vi "Arm Main.vi"() -> ()   [LabVIEW 2013]
doc: "This example shows how to move a motor connected to an encoder and a wheel, and then read information about the system from an encoder.\n\nThis is an example of how to use feedback (from the encoder) to create an open loop system. If some control method was used, for example using PID, a closed loop system could be created."
uses:
  <vilib>/Rock Robotics/WPI/DriverStation/WPI_DriverStationRobotMode2.ctl
  Robot Global Data.vi
panel:
  in  "Increment Down":dbl=-8.0
  in  "Increment Up":dbl=5.0
  in  "Incremented Angle":dbl=180.0
  in  "Biased Voltage":dbl=-0.5
  in  "Motor Upper Limit":dbl format="%#_13g"
  in  "Motor Lower Limit":dbl=-0.55 format="%#_13g"
  out "Arm Angle":dbl(graph)=177.5123200166945
  out "Motor Output":dbl(graph)
  in  "Arm Gain":dbl=0.01
  out "Arm Angle (deg)":dbl(knob)=177.5123200166945 scale=0.0..360.0 scale format="%#_3g"
  # "Output information."
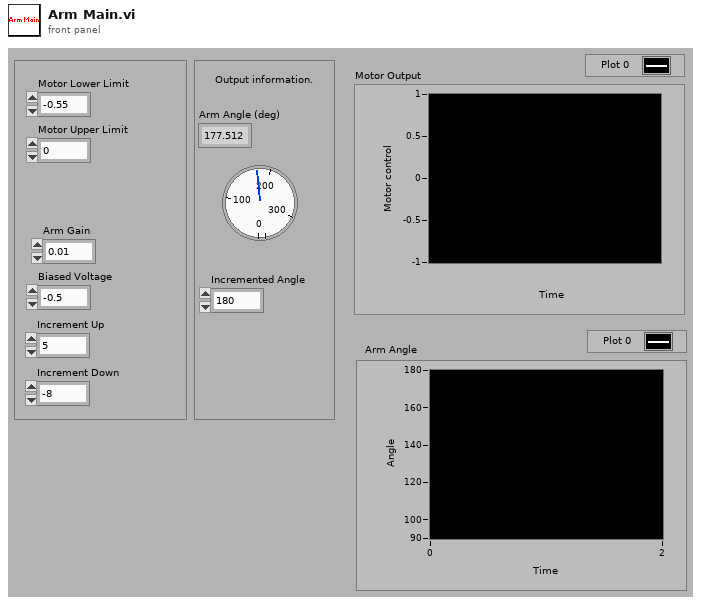
[diagram p1: front panel]
types:
  T1 = typedef "WPI_DriverStationRobotMode2.ctl" = enum16{"Autonomous Disabled", "Autonomous Enabled", "Teleop Disabled", "Teleop Enabled", "Timeout", "Finish", "Test Disabled", "Test Enabled"}
  T2 = cluster{"Axes":cluster{"LS X":dbl, "LS Y":dbl, "Triggers":dbl, "RS X":dbl, "RS Y":dbl}, "Buttons":cluster{"LT":bool, "RT":bool, "A":bool, "B":bool, "X":bool, "Y":bool, "LB":bool, "RB":bool, "Back":bool, "Start":bool, "LS":bool, "RS":bool}, "Buttons Just Pushed":cluster{"LT":bool, "RT":bool, "A":bool, "B":bool, "X":bool, "Y":bool, "LB":bool, "RB":bool, "Back":bool, "Start":bool, "LS":bool, "RS":bool}}
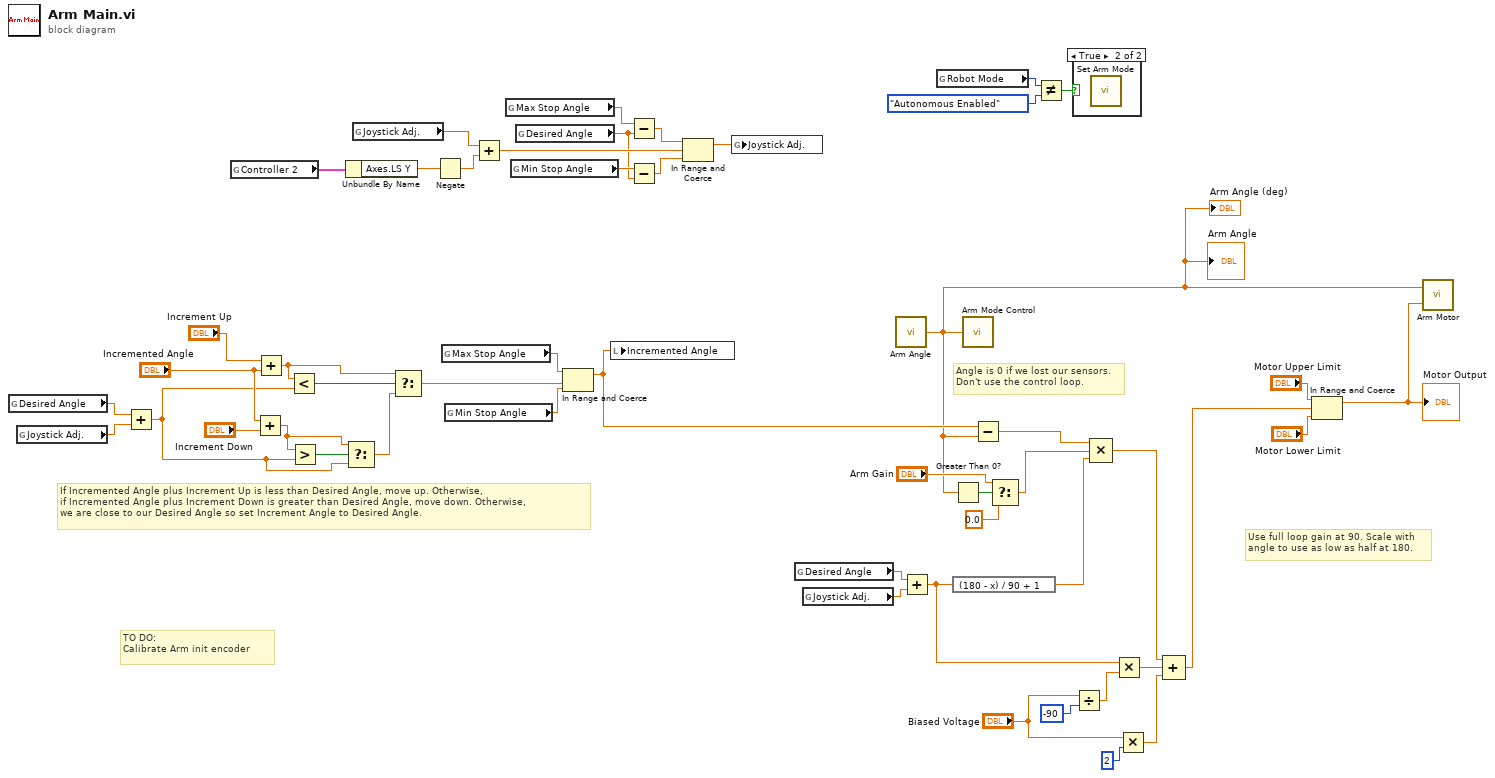
[diagram p0: block diagram]
diagram:
  # "Use full loop gain at 90. Scale with \nangle to use as low as half at 180."
  # "Angle is 0 if we lost our sensors.\nDon't use the control loop."
  # "If Incremented Angle plus Increment Up is less than Desired Angle, move up. Otherwise,\nif Incremented Angle plus Increment Down is greater than Desired Angle, move down. Otherwise,\nwe are close to our Desired Angle so set Increment Angle to Desired Angle."
  # "TO DO:\nCalibrate Arm init encoder"
  n1 = global read "Robot Global Data.vi" "Desired Angle"() -> (w28:dbl)
  n2 = global read "Robot Global Data.vi" "Joystick Adj."() -> (w26:dbl)
  n3 = Add(x=w28, y=w26) -> (x+y=w27:dbl)
  n4 = global read "Robot Global Data.vi" "Controller 2"() -> (w14:T2)
  n5 = Add(x="Incremented Angle", y="Increment Down") -> (x+y=w38:dbl)
  n6 = Add(x="Increment Up", y="Incremented Angle") -> (x+y=w40:dbl)
  n7 = Less?(x=w40, y=w27) -> (x < y?=w41:bool)
  n8 = Greater?(x=w38, y=w27) -> (0:w39:bool)
  n9 = Unbundle By Name(w14) -> ("Axes.LS Y"=w45:dbl)
  n10 = Select(t=w38, s=w39, f=w27) -> (s? t:f=w37:dbl)
  n11 = global read "Robot Global Data.vi" "Joystick Adj."() -> (w25:dbl)
  n12 = Select(t=w40, s=w41, f=w37) -> (s? t:f=w34:dbl)
  n13 = Negate(x=w45) -> (-x=w32:dbl)
  n14 = global read "Robot Global Data.vi" "Max Stop Angle"() -> (w36:dbl)
  n15 = global read "Robot Global Data.vi" "Min Stop Angle"() -> (w35:dbl)
  n16 = Add(x=w25, y=w32) -> (x+y=w23:dbl)
  n17 = global read "Robot Global Data.vi" "Max Stop Angle"() -> (w22:dbl)
  n18 = global read "Robot Global Data.vi" "Min Stop Angle"() -> (w19:dbl)
  n19 = global read "Robot Global Data.vi" "Desired Angle"() -> (w18:dbl)
  n20 = In Range and Coerce(upper limit=w36, x=w34, lower limit=w35) -> (coerced(x)=w33:dbl)  [unwired: 1 out]
  n21 = local write "Incremented Angle"(w33) -> ()
  n22 = Subtract(x=w22, y=w18) -> (x-y=w21:dbl)
  n23 = Subtract(x=w19, y=w18) -> (x-y=w20:dbl)
  n24 = In Range and Coerce(upper limit=w21, x=w23, lower limit=w20) -> (coerced(x)=w24:dbl)  [unwired: 1 out]
  n25 = global write "Robot Global Data.vi" "Joystick Adj."(w24) -> ()
  n26 = global read "Robot Global Data.vi" "Desired Angle"() -> (w16:dbl)
  n27 = global read "Robot Global Data.vi" "Joystick Adj."() -> (w17:dbl)
  n28 = call "Arm Angle.vi"() -> ("Angle"=w1:dbl)  [unwired: 1 in]
  "Arm Angle (deg)" <- w1
  "Arm Angle" <- w1
  n29 = Add(x=w16, y=w17) -> (x+y=w8:dbl)
  n30 = global read "Robot Global Data.vi" "Robot Mode"() -> (w31:T1)
  n31 = Greater Than 0?(x=w1) -> (x > 0?=w6:bool)
  n32 = expression code="(180 - x) / 90 + 1"(w8) -> (w13:dbl)
  n33 = call "Arm Mode Control.vi"("Current Angle"=w1) -> ()  [unwired: 1 in]
  n34 = Subtract(x=w33, y=w1) -> (x-y=w15:dbl)
  n35 = Select(t="Arm Gain", s=w6, f=0.0) -> (s? t:f=w3:dbl)
  n36 = Not Equal?(x=w31, y=WPI_DriverStationRobotMode2."Autonomous Enabled" ("Robot Mode")) -> (x != y?=w29:bool)
  n37 = case shown="True" w29 {
    frame False {
    }
    frame True {
      n38 = call "Set Arm Mode.vi"() -> ()  [unwired: 1 in]
    }
  }
  n39 = Divide(x="Biased Voltage", y=-90) -> (x/y=w7:dbl)
  n40 = Compound Arithmetic op=MULTIPLY(w15, w3, w13) -> (w10:dbl)
  n41 = Multiply(x=w8, y=w7) -> (x*y=w11:dbl)
  n42 = Multiply(x="Biased Voltage", y=2) -> (x*y=w12:dbl)
  n43 = Compound Arithmetic op=ADD(w10, w11, w12) -> (w9:dbl)
  n44 = In Range and Coerce(upper limit="Motor Upper Limit", x=w9, lower limit="Motor Lower Limit") -> (coerced(x)=w2:dbl)  [unwired: 1 out]
  "Motor Output" <- w2
  n45 = call "Arm Motor.vi"("Motor input"=w2, "Current angle (deg)"=w1) -> ()  [unwired: 1 in]
